vi "ATM Menu Handler.vi"(8 "error in (no error)":errorcluster, 11 "Menu State":string) -> (0 "error out":errorcluster, 3 "Menu Items":string[](array[string]))   [LabVIEW 2011]
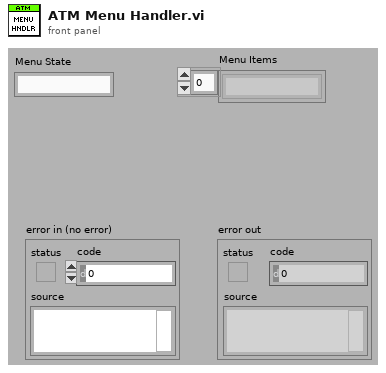
[diagram p1: front panel]
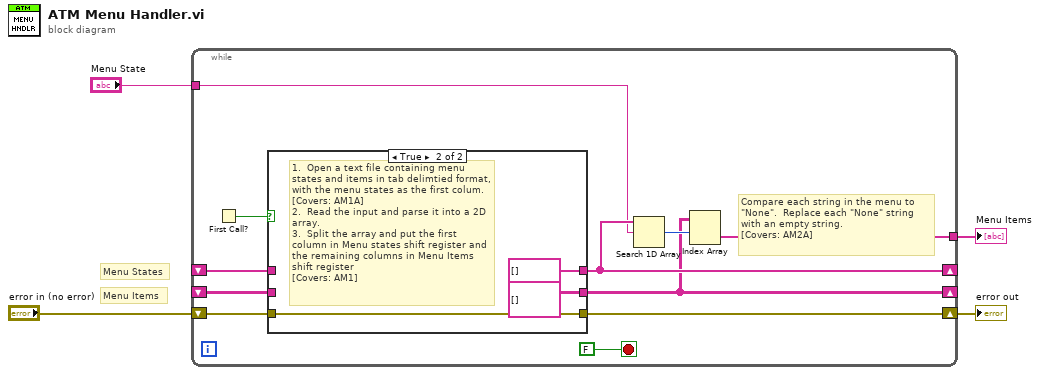
[diagram p0: block diagram]
diagram:
  # "Menu Items"
  # "Menu States"
  n1 = while {
    shift-right: [w13] -> w3
    shift-left: "error in (no error)" -> [w14]
    shift-right: [w9] -> _
    shift-left: _ -> [w11]
    shift-right: [w6] -> _
    shift-left: _ -> [w10]
    tunnel: "Menu State" -> [w8]
    tunnel: [w5] -> w1
    stop <- FALSE stop-if-true
    # "Compare each string in the menu to\n\"None\".  Replace each \"None\" string\nwith an empty string.\n[Covers: AM2A]"
    n2 = First Call?() -> (First Call?: T/F=w15:bool)
    n3 = case shown="True" w15 {
      tunnel: w14 -> [w16 w21]
      tunnel: [w16 w21] -> w13
      tunnel: [w18 string[] [] ("Parameters")] -> w9
      tunnel: [w17 string[][] [] ("Parameters")] -> w6
      tunnel: w11 -> [w18 _]
      tunnel: w10 -> [w17 _]
      frame False {
      }
      frame True {
        # "1.  Open a text file containing menu states and items in tab delimtied format,\nwith the menu states as the first colum.\n[Covers: AM1A]\n2.  Read the input and parse it into a 2D array.\n3.  Split the array and put the first column in Menu states shift register and the remaining columns in Menu Items shift register\n[Covers: AM1]"
      }
    }
    n4 = Search 1D Array(1D array=w9, element=w8) -> (index of element=w7:i32)  [unwired: 1 in]
    n5 = Index Array(array=w6, index (row)=w7) -> (element=w5:string[])  [unwired: 1 in]
  }
  "error out" <- w3
  "Menu Items" <- w1
